vi "main_time_control.vi"(9 "Running?":refnum<vi>, 10 "Endtime":refnum<vi>, 11 "Starttime":refnum<vi>) -> ()   [LabVIEW 2019]
uses:
  lib/libSimulationControl/libSimulationControl.lvlib
panel:
  # "*******************************************************************\nBiogas Plant Control\n\nAuthor: Paul Zügel\nGCSC-Frankfurt am Main 2020\n\n*******************************************************************"
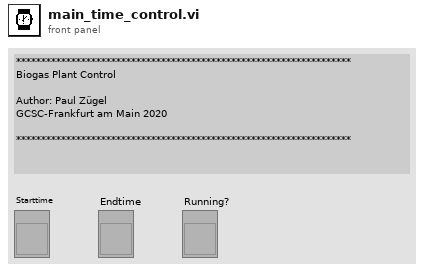
[diagram p1: front panel]
types:
  T1 = enum8{"Enabled", "Disabled", "Disabled and Grayed Out"}
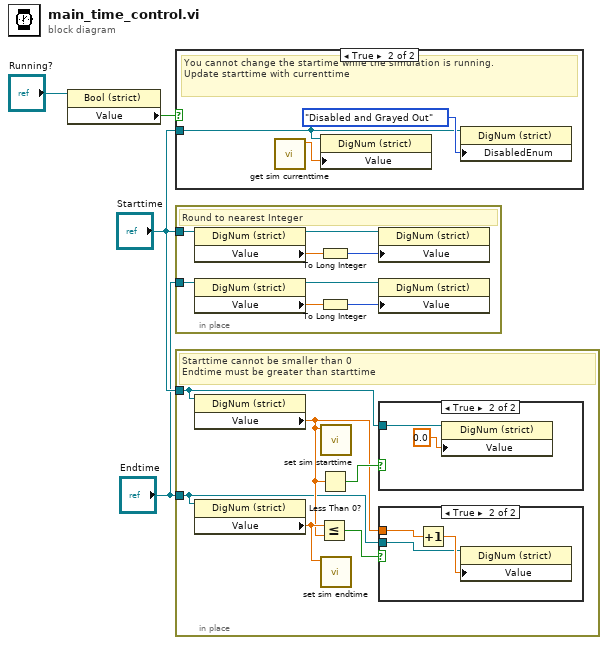
[diagram p0: block diagram]
diagram:
  n1 = property on="Property Node" class="Bool (strict)"(reference="Running?") -> ("Value"=w3:bool)  [unwired: 1 in, 2 out]
  n2 = case shown="True" w3 {
    tunnel: "Starttime" -> [_ w6]
    frame False {
      # "Disable starttime when simulatiuon is running"
    }
    frame True {
      # "You cannot change the startime while the simulation is running.\nUpdate starttime with currenttime"
      n3 = call "get sim currenttime.vi"() -> ("current_time"=w5:dbl)  [unwired: 10 in, 1 out]
      n4 = property on="Property Node" class="DigNum (strict)"(reference=w6, "Value"=w5) -> ()  [unwired: 1 in, 2 out]
      n5 = property class="DigNum (strict)"(reference=w6, "DisabledEnum"=T1."Disabled and Grayed Out" ("Disabled")) -> ()  [unwired: 1 in, 2 out]
    }
  }
  n6 = in-place {
    in-place-border: "Starttime" -> [w11]
    in-place-border: "Endtime" -> [w10]
    # "Round to nearest Integer"
    n7 = property on="Property Node" class="DigNum (strict)"(reference=w11) -> (reference out=w9:refnum<vi>, "Value"=w15:dbl)  [unwired: 1 in, 1 out]
    n8 = property on="Property Node" class="DigNum (strict)"(reference=w10) -> (reference out=w8:refnum<vi>, "Value"=w13:dbl)  [unwired: 1 in, 1 out]
    n9 = To Long Integer(number=w15) -> (32bit integer=w14:i32)
    n10 = To Long Integer(number=w13) -> (32bit integer=w12:i32)
    n11 = property on="Property Node" class="DigNum (strict)"(reference=w9, "Value"=w14) -> ()  [unwired: 1 in, 2 out]
    n12 = property on="Property Node" class="DigNum (strict)"(reference=w8, "Value"=w12) -> ()  [unwired: 1 in, 2 out]
  }
  n13 = in-place {
    in-place-border: "Starttime" -> [w17]
    in-place-border: "Endtime" -> [w16]
    # "Starttime cannot be smaller than 0\nEndtime must be greater than starttime"
    n14 = property on="Property Node" class="DigNum (strict)"(reference=w17) -> ("Value"=w18:dbl)  [unwired: 1 in, 2 out]
    n15 = property on="Property Node" class="DigNum (strict)"(reference=w16) -> ("Value"=w19:dbl)  [unwired: 1 in, 2 out]
    n16 = Less Or Equal?(x=w19, y=w18) -> (x <= y?=w20:bool)
    n17 = Less Than 0?(x=w18) -> (x < 0?=w21:bool)
    n18 = call "set sim starttime.vi"("time"=w18) -> ()  [unwired: 10 in, 1 out]
    n19 = call "set sim endtime.vi"("time"=w19) -> ()  [unwired: 10 in, 1 out]
    n20 = case shown="True" w21 {
      tunnel: w17 -> [_ w22]
      frame False {
      }
      frame True {
        n21 = property on="Property Node" class="DigNum (strict)"(reference=w22, "Value"=0.0 ("Starttime")) -> ()  [unwired: 1 in, 2 out]
      }
    }
    n22 = case shown="True" w20 {
      tunnel: w16 -> [_ w25]
      tunnel: w18 -> [_ w24]
      frame False {
      }
      frame True {
        n23 = Increment(x=w24) -> (x+1=w26:dbl)
        n24 = property on="Property Node" class="DigNum (strict)"(reference=w25, "Value"=w26) -> ()  [unwired: 1 in, 2 out]
      }
    }
  }
